vi "4.3.1.vi"() -> ()   [LabVIEW 2017]
panel:
  in  "Amplitude 2":dbl(slide) scale=0.0..10.0
  in  "Amplitude 1":dbl(slide) scale=0.0..10.0
  out "Waveform Graph":dynamicdata(graph)
  in  "stop":bool
  in  "Frequency 2":dbl
  in  "Frequency 1":dbl
  in  "Phase 2":dbl
  in  "Phase 1":dbl
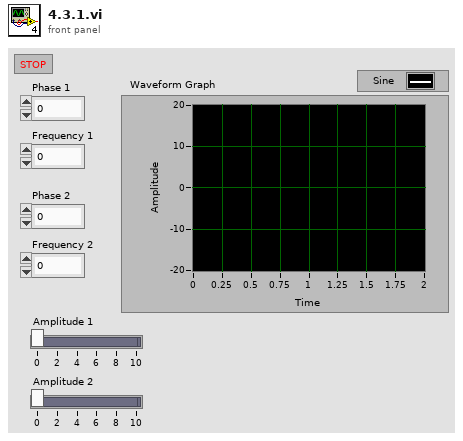
[diagram p1: front panel]
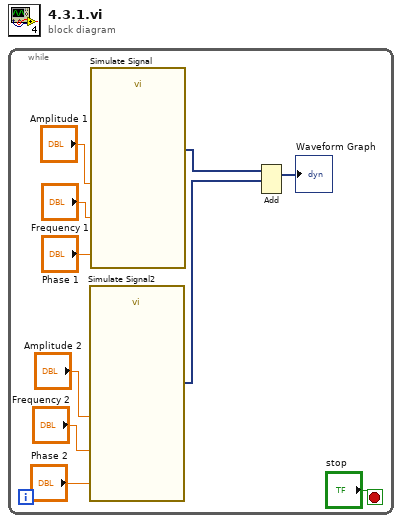
[diagram p0: block diagram]
diagram:
  n1 = while {
    stop <- "stop" stop-if-true
    n2 = call "Simulate Signal2"("Frequency"="Frequency 2", "Amplitude"="Amplitude 2", "Phase"="Phase 2") -> ("Sine"=w5:dynamicdata)  [unwired: 11 in, 1 out]
    n3 = call "Simulate Signal"("Frequency"="Frequency 1", "Amplitude"="Amplitude 1", "Phase"="Phase 1") -> ("Sine"=w4:dynamicdata)  [unwired: 11 in, 1 out]
    n4 = Add(1:w5, 2:w4) -> (0:→"Waveform Graph":dynamicdata)  [unwired: 1 in, 1 out]
  }
